vi "Autonomous State global.vi"() -> ()   [LabVIEW 2015]
uses:
  Autonomous Play State.ctl
  Autonomous Commands/Autonomous Command Names.ctl
panel:
  out "Autonomous Execution State":T1
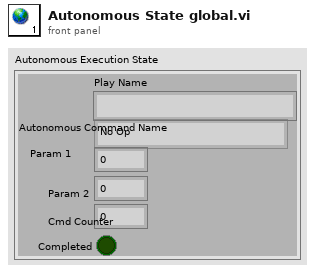
[diagram p1: front panel]
types:
  T1 = typedef "Autonomous Play State.ctl" = cluster{"Play Name":string, "Autonomous Command Name":T2, "Param 1":dbl, "Param 2":dbl, "Cmd Counter":i32, "Completed":bool}
  T2 = typedef "Autonomous Command Names.ctl" = enum16{"No Op"}
diagram:
